vi "Get Test Case Item ID.vi"(8 "error in (no error)":errorcluster, 10 "Test Case":string, 11 "Icon Decorator V2 In":refnum<class "Icon Decorator V2.lvclass">) -> (0 "error out":errorcluster, 2 "ObjectItem":T1, 3 "Icon Decorator V2 Out":refnum<class "Icon Decorator V2.lvclass">)   [LabVIEW 2020, in "Icon Decorator V2.lvclass"]
uses:
  Icon Decorator V2.lvclass
  <resource>/Framework/Providers/API/ItemRef.ctl
  Icon Decorator V2.lvclass/Icon Decorator V2.ctl
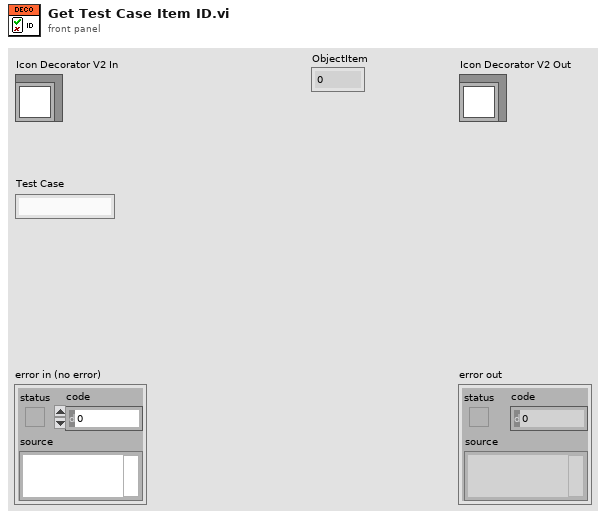
[diagram p1: front panel]
types:
  T1 = typedef "ItemRef.ctl" = u64
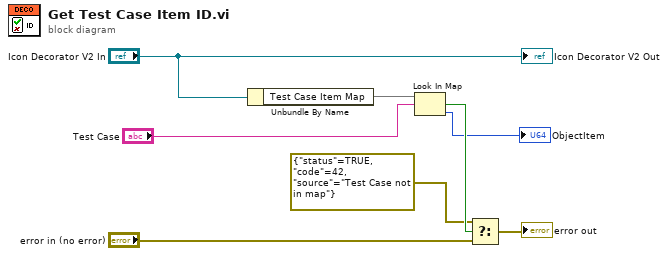
[diagram p0: block diagram]
diagram:
  n1 = Unbundle By Name("Icon Decorator V2 In") -> ("Test Case Item Map"=w6:map{string, T1})
  n2 = Look In Map(map=w6, key="Test Case") -> (key not found?=w3:bool, value=→"ObjectItem":T1)  [unwired: 1 in]
  n3 = Select(t=errorcluster {"status"=TRUE, "code"=42, "source"="Test Case not in map"}, s=w3, f="error in (no error)") -> (s? t:f=→"error out":errorcluster)
  "Icon Decorator V2 Out" <- "Icon Decorator V2 In"
